vi "Read TestDataMgr Handle.vi"(8 "error in (no error)":errorcluster, 11 "STDF File Parser in":refnum<class "STDF File Parser.lvclass">) -> (0 "error out":errorcluster, 2 "Session Handle":T1, 3 "STDF File Parser out":refnum<class "STDF File Parser.lvclass">)   [LabVIEW 2018, in "STDF File Parser.lvclass"]
uses:
  STDF File Parser.lvclass
  TestDataMgr/Typedefs/Session Handle.ctl
  TestDataMgr/TestDataMgr.lvclass
  STDF File Parser.lvclass/STDF File Parser.ctl
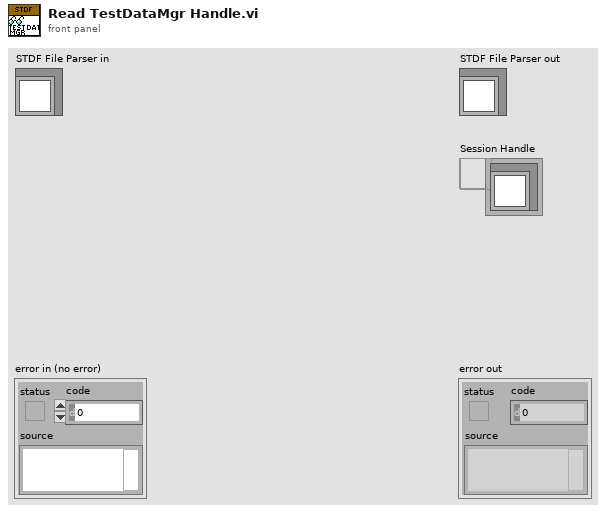
[diagram p1: front panel]
types:
  T1 = typedef "TestDataMgr.lvclass/Session Handle.ctl" = refnum<data-value>
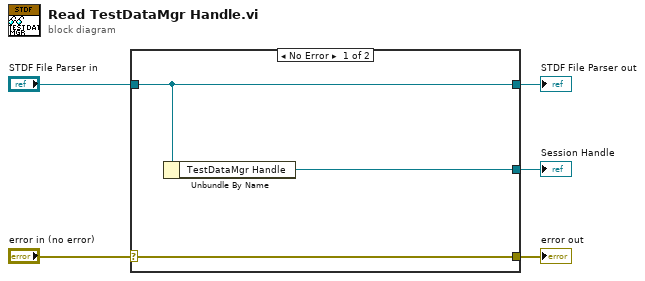
[diagram p0: block diagram]
diagram:
  n1 = case shown="No Error" "error in (no error)" {
    selector: "error in (no error)" -> [w8 w9]
    tunnel: [w8 w9] -> w4
    tunnel: [w7 w10] -> w2
    tunnel: "STDF File Parser in" -> [w7 w10]
    tunnel: [w6 _] -> w1
    frame No Error {
      n2 = Unbundle By Name(w7) -> ("TestDataMgr Handle"=w6:T1)
    }
    frame Error {
    }
  }
  "error out" <- w4
  "STDF File Parser out" <- w2
  "Session Handle" <- w1
